vi "FPGA Audio Configure (SubVI).vi"(8 "error in (no error)":errorcluster, 9 "Read Rate (Hz)":dbl=10.0, 10 "Audio Sample Rate (Hz)":dbl=44101.0, 11 "Refnum in":refnum<k20>) -> (0 "error out":errorcluster, 1 "Required loop period (ms)":u32, 2 "Audio dt (ms)":dbl, 3 "Refnum out":refnum<k20>)   [LabVIEW 2016]
uses:
  <vilib>/Utility/error.llb/Error Cluster From Error Code.vi
  <vilib>/rvi/errors/niLvFpgaAdjustHostInterfaceError.vi
  <vilib>/rvi/interface/common/niFpgaWaitOnOcc.vi
  <vilib>/FPGAPlugInAG/Dynamic/niLvFpga_Run_Dynamic.vi
  <vilib>/rvi/interface/nirviReadWriteControl/nirviReadWriteControl.xnode
  <vilib>/rvi/interface/nirviMethod/nirviMethod.xnode
  <vilib>/rvi/errors/niLvFpgaMergeErrorWithErrorCode.vi
  NiFpgaLv.dll
  <vilib>/rvi/interface/Simulation/niFpgaSimulationCallBeginRW.vi
  <vilib>/FPGAPlugInAG/Dynamic/niLvFpga_ConfigureFifo_Dynamic.vi
  <vilib>/FPGAPlugInAG/Dynamic/niLvFpga_StartFifo_Dynamic.vi
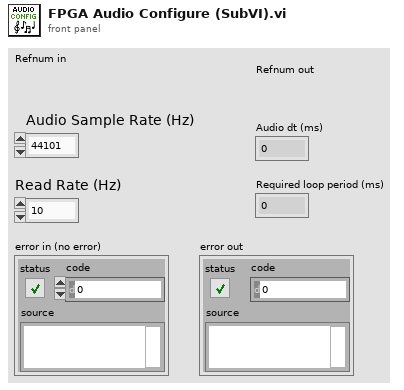
[diagram p1: front panel]
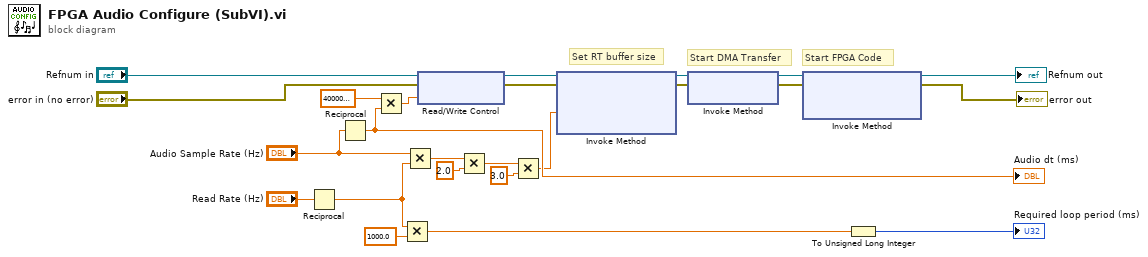
[diagram p0: block diagram]
diagram:
  # "Start FPGA Code"
  # "Start DMA Transfer"
  # "Set RT buffer size"
  n1 = Reciprocal(x="Read Rate (Hz)") -> (1/x=w10:dbl)
  n2 = Reciprocal(x="Audio Sample Rate (Hz)") -> (1/x=w23:dbl)
  "Audio dt (ms)" <- w23
  n3 = Multiply(x=40000000.0 ("y"), y=w23) -> (x*y=w22:dbl)
  n4 = Multiply(x=w10, y=1000.0) -> (x*y=w9:dbl)
  n5 = Multiply(x="Audio Sample Rate (Hz)", y=w10) -> (x*y=w11:dbl)
  n6 = xnode "Read/Write Control"("FPGA VI Reference In"="Refnum in", "error in"="error in (no error)", "Count(Ticks)"=w22) -> ("FPGA VI Reference Out"=w19:refnum<k20>, "error out"=w17:errorcluster)
  n7 = Multiply(x=w11, y=2.0) -> (x*y=w13:dbl)
  n8 = Multiply(x=w13, y=3.0) -> (x*y=w15:dbl)
  n9 = xnode "Invoke Method"("FPGA VI Reference In"=w19, "error in"=w17, "Requested Depth"=w15) -> ("FPGA VI Reference Out"=w1:refnum<k20>, "error out"=w6:errorcluster)  [unwired: 1 out]
  n10 = xnode "Invoke Method"("FPGA VI Reference In"=w1, "error in"=w6) -> ("FPGA VI Reference Out"=w3:refnum<k20>, "error out"=w4:errorcluster)
  n11 = xnode "Invoke Method"("FPGA VI Reference In"=w3, "error in"=w4) -> ("FPGA VI Reference Out"=→"Refnum out":refnum<k20>, "error out"=→"error out":errorcluster)  [unwired: 1 in]
  n12 = To Unsigned Long Integer(number=w9) -> (unsigned 32bit integer=→"Required loop period (ms)":u32)
